vi "FGV.vi"(9 "FilteredVisionData":T1, 10 "?":T3, 11 "Write Average":T2) -> (3 "FilteredVisionData 2":T1)   [LabVIEW 2018, in "Vision.lvlib" / "Vision.lvclass"]
uses:
  Vision.lvclass
  Controls/FGVData.ctl
  Controls/FGVEnum.ctl
  FilteredVisionData.ctl
panel:
  out "Write Average 2":T2
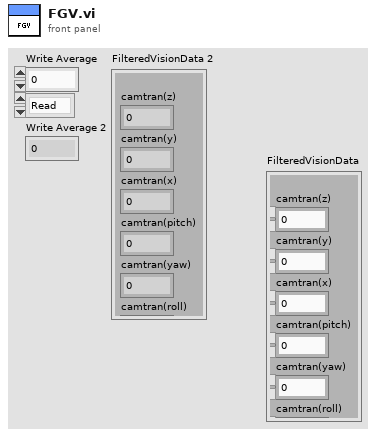
[diagram p1: front panel]
types:
  T1 = typedef "Vision.lvlib/Vision.lvclass/FilteredVisionData.ctl" = cluster{"camtran(z)":dbl, "camtran(x)":dbl, "camtran(pitch)":dbl, "camtran(y)":dbl, "camtran(roll)":dbl, "camtran(yaw)":dbl}
  T2 = typedef "Vision.lvlib/Vision.lvclass/FGVData.ctl" = dbl
  T3 = typedef "Vision.lvlib/Vision.lvclass/FGVEnum.ctl" = enum16{"Read", "Write"}
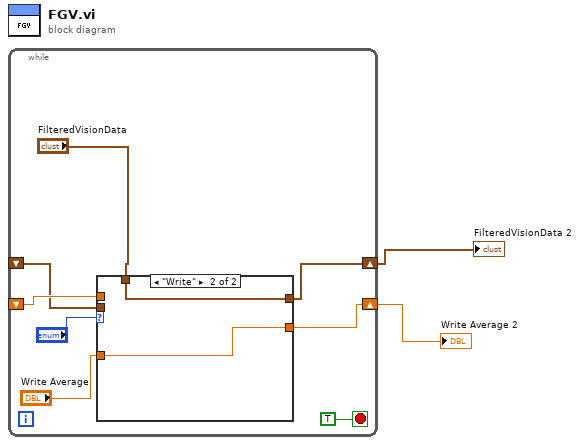
[diagram p0: block diagram]
diagram:
  n1 = while {
    shift-right: [w7] -> w2
    shift-left: _ -> [w8]
    shift-right: [w4] -> w1
    shift-left: _ -> [w3]
    stop <- TRUE stop-if-true
    n2 = case shown="\"Write\"" "?" {
      tunnel: w8 -> [w12 _]
      tunnel: [w12 w14] -> w7
      tunnel: "Write Average" -> [_ w14]
      tunnel: "FilteredVisionData" -> [_ w13]
      tunnel: [w11 w13] -> w4
      tunnel: w3 -> [w11 _]
      frame "Read", Default {
      }
      frame "Write" {
      }
    }
  }
  "Write Average 2" <- w2
  "FilteredVisionData 2" <- w1
